vi "Actor Core.vi"(8 "error in":errorcluster, 11 "Create Test Node View in":refnum<class "Edit Test Node View.lvclass">) -> (0 "error out":errorcluster, 3 "Actor out":refnum<class "Actor.lvclass">)   [LabVIEW 2013, in "Edit Test Node View.lvlib" / "Edit Test Node View.lvclass"]
doc: "(<B>Filename</B>: Actor Framework.lvlib:Actor.lvclass:Actor Core.vi)\n\nReceives messages to the actor, reacts to them, and initiates any error handling that may shut the actor down.\n\nDescendant classes may override this VI to append parallel tasks for the actor to complete while it handles messages. Overrides use the Call Parent Method node."
uses:
  Edit Test Node View.lvclass
  <vilib>/ActorFramework/Actor/Actor.lvclass
  Resources/UI Controls/Textbox.ctl
  <vilib>/ActorFramework/Actor/Actor.lvclass/Actor.ctl
  <vilib>/ActorFrameworkMVC/View Actor/View Actor.lvclass
  <vilib>/ActorFramework/Message Enqueuer/Message Enqueuer.lvclass/Message Enqueuer.ctl
  Edit Test Node View.lvclass/Edit Test Node View.ctl
  Models/Edit Test Node Model Messages/Set Item Configurations Msg/Set Item Configurations Msg.lvclass/Set Item Configurations Msg.ctl
  <vilib>/Utility/miscctls.llb/LVPositionTypeDef.ctl
  <vilib>/ActorFrameworkMVC/UI Controller Messages/Move Subpanel Msg/Move Subpanel Msg.lvclass/Move Subpanel Msg.ctl
  <vilib>/ActorFrameworkMVC/UI Controller Messages/Insert Subpanel Msg/Insert Subpanel Msg.lvclass/Insert Subpanel Msg.ctl
  <vilib>/ActorFramework/Message Enqueuer/Init from Existing Queue.vi
  <vilib>/ActorFramework/Message Enqueuer/Enqueue.vi
  <vilib>/ActorFramework/Message Priority Queue/Priority Enqueue.vi
  <vilib>/ActorFramework/Message Enqueuer/Message Enqueuer.lvclass
  Models/Edit Test Node Model Messages/Set Item Configurations Msg/Set Item Configurations Msg.lvclass
  Models/Edit Test Node Model Messages/Load Test Node Msg/Load Test Node Msg.lvclass
  Models/Edit Test Node Model Messages/Save Test Node Msg/Save Test Node Msg.lvclass
  <vilib>/ActorFrameworkMVC/UI Controller Messages/Move Subpanel Msg/Move Subpanel Msg.lvclass
  <vilib>/ActorFrameworkMVC/UI Controller Messages/Insert Subpanel Msg/Insert Subpanel Msg.lvclass
  Models/Test Node Model Messages/Preview Test Node Msg/Preview Test Node Msg.lvclass
  Models/Test Node Model Messages/Update Tiles Info Msg/Update Tiles Info Msg.lvclass
  Models/Test Node Model Messages/Update Previous Button Visibility Msg/Update Previous Button Visibility Msg.lvclass
  Models/Test Node Model Messages/Update Next Button Visibility Msg/Update Next Button Visibility Msg.lvclass
  Common/File IO/File IO.lvlib
  <vilib>/ActorFrameworkMVC/View Actor Messages/Get Model Enqueuer Msg/Get Model Enqueuer Msg.lvclass
  <vilib>/ActorFrameworkMVC/UI Controller Messages/Get Model Actor Enqueuer Msg/Get Model Actor Enqueuer Msg.lvclass
panel:
  in  "Cancel":bool
  in  "Save":bool
  out "Tab Control":enum32{"Basic Info"}(tab)
  in  "Node Description":string caption="测试节点描述："
  in  "Node Name":string caption="测试节点名称："
  in  "Node Abbreviation":string caption="测试节点英文简写："
  in  "Node Type":u16(ring) caption="测试节点类型：" items=["模拟电压", "模拟电流", "数字", "RS232", "RS485"]
  in  "Node MAC":T1 caption="测试节点MAC"
  # "编辑测试节点"
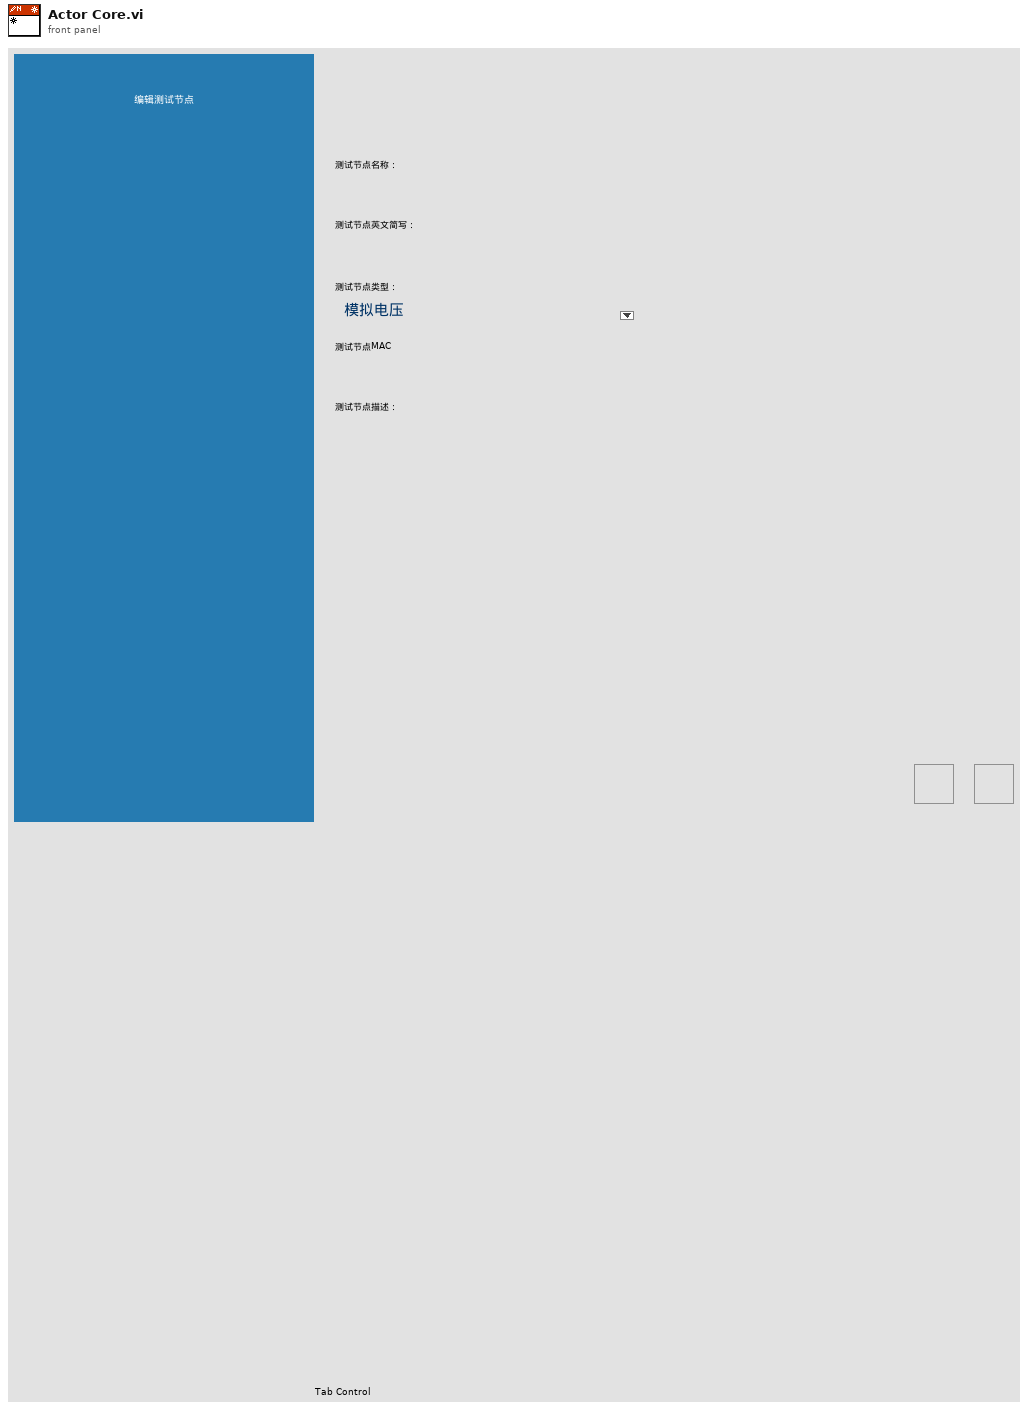
[diagram p1: front panel]
types:
  T1 = typedef "Textbox.ctl" = string
  T2 = typedef "Edit Test Node View.lvlib/Edit Test Node View.lvclass/Events.ctl" = cluster{"Reinitialize All":refnum<user-event>}
  T3 = typedef "LVPositionTypeDef.ctl" = cluster{"Left":i32, "Top":i32}
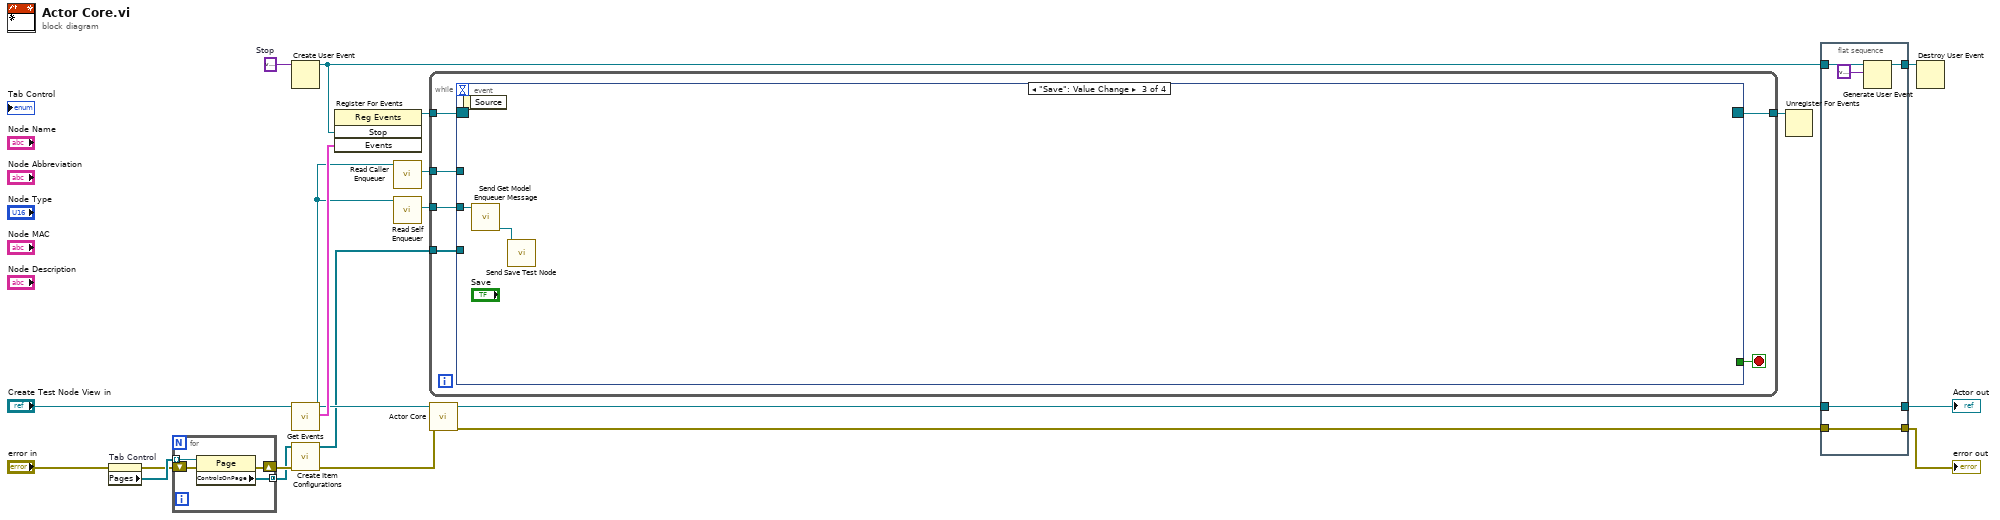
[diagram p0: block diagram]
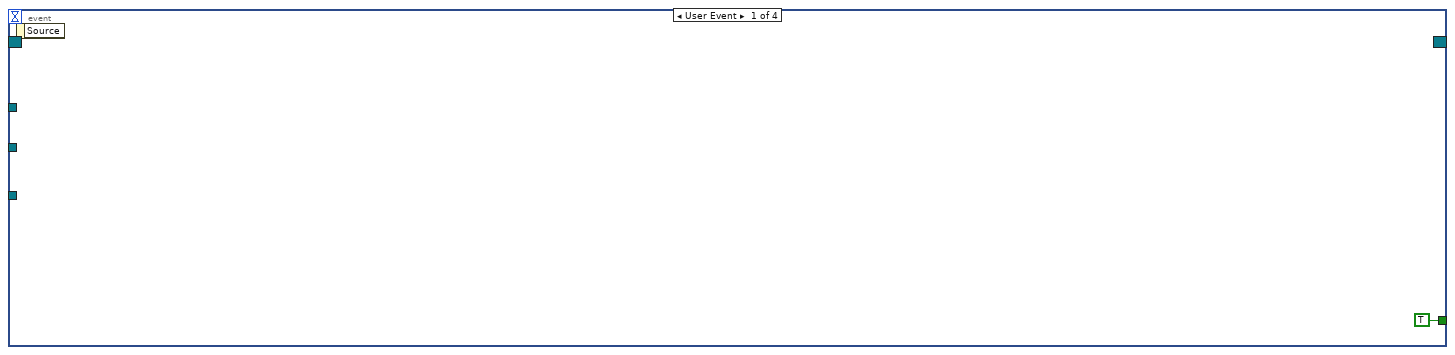
[diagram p2: hidden frame]
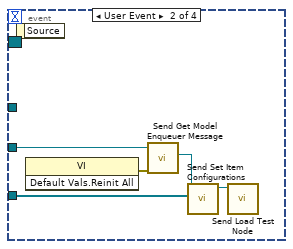
[diagram p3: hidden frame]
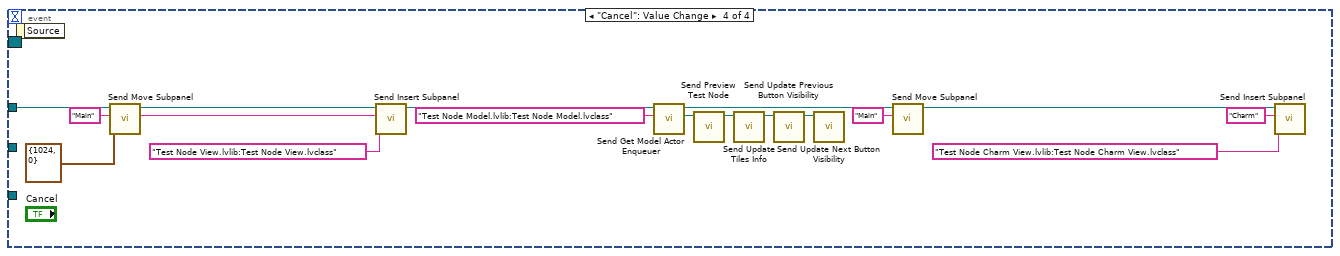
[diagram p4: hidden frame]
diagram:
  w21 = variant  # Stop
  n1 = property on="Tab Control" class="TabCtl (strict)"(error in="error in") -> (error out=w10:errorcluster, "Pages"=w11:refnum<vi>[])  [unwired: 1 in, 1 out]
  n2 = for {
    tunnel: w11 -> [w25] mode=indexing
    tunnel: [w24] -> w8 mode=concatenating
    shift-right: [w22] -> w9
    shift-left: w10 -> [w23]
    n3 = property class="Page"(reference=w25, error in=w23) -> (error out=w22:errorcluster, "ControlsOnPage"=w24:refnum<vi>[])  [unwired: 1 out]
  }
  n4 = Create User Event(user event datatype=w21) -> (user event=w14:refnum<user-event>)  [unwired: 1 in, 1 out]
  n5 = call "Get Events.vi"("Create Test Node View in"="Create Test Node View in") -> ("Events"=w13:T2, "Create Test Node View out"=w4:refnum<class "Edit Test Node View.lvclass">)  [unwired: 9 in]
  n6 = call "Create Item Configurations.vi"("error in (no error)"=w9, "Controls References"=w8) -> ("error out"=w3:errorcluster, "Item Configurations"=w1:refnum<class "Item Configuration.lvclass">[])  [unwired: 8 in]
  n7 = register-events(w14, w13) -> (reference out=w15:refnum<event-registration>)  [unwired: 2 in, 1 out]
  n8 = call <vilib>:"Read Caller Enqueuer.vi"("Actor"=w4) -> ("Caller Enqueuer"=w6:refnum<class "Message Enqueuer.lvclass">)  [unwired: 10 in]
  n9 = call <vilib>:"Read Self Enqueuer.vi"("Actor"=w4) -> ("Self Enqueuer"=w5:refnum<class "Message Enqueuer.lvclass">)  [unwired: 10 in]
  n10 = while {
    tunnel: [w31] -> w12
    tunnel: w15 -> [w29]
    tunnel: w6 -> [w28]
    tunnel: w5 -> [w27]
    tunnel: w1 -> [w26]
    stop <- w30 stop-if-true
    n11 = event shown="[2] \"Save\": Value Change" {
      selector: w29 -> [_ _ _ _]
      dyn-events: [_ _ _ _] -> w31
      timeout: _ -> [_ _ _ _]
      tunnel: [TRUE _ _ _] -> w30
      tunnel: w28 -> [_ _ _ w41]
      tunnel: w27 -> [_ w34 w38 _]
      tunnel: w26 -> [_ w33 _ _]
      event User Event {
        n12 = event-data() -> ()  [unwired: 1 in, 1 out]
      }
      event User Event {
        n13 = event-data() -> ()  [unwired: 1 in, 1 out]
        n14 = invoke class="VI" method="Default Vals.Reinit All"() -> (error out=w37:errorcluster)  [unwired: 3 in, 2 out]
        n15 = call <vilib>:"Send Get Model Enqueuer Message.vi"("error in (no error)"=w37, "Message Enqueuer in"=w34) -> ("Reply"=w36:refnum<class "Message Enqueuer.lvclass">)  [unwired: 6 in, 3 out]
        n16 = call "Send Set Item Configurations.vi"("Item Configurations"=w33, "Message Enqueuer"=w36) -> ("Message Enqueuer out"=w35:refnum<class "Message Enqueuer.lvclass">)  [unwired: 8 in, 1 out]
        n17 = call "Send Load Test Node.vi"("Message Enqueuer"=w35) -> ()  [unwired: 9 in, 2 out]
      }
      event "Save": Value Change {
        n18 = event-data() -> ()  [unwired: 1 in, 1 out]
        n19 = call <vilib>:"Send Get Model Enqueuer Message.vi"("Message Enqueuer in"=w38) -> ("Reply"=w39:refnum<class "Message Enqueuer.lvclass">)  [unwired: 7 in, 3 out]
        n20 = call "Send Save Test Node.vi"("Message Enqueuer"=w39) -> ()  [unwired: 9 in, 2 out]
      }
      event "Cancel": Value Change {
        w52 = "Main" ("Subpanel Name")
        n21 = event-data() -> ()  [unwired: 1 in, 1 out]
        n22 = call <vilib>:"Send Move Subpanel.vi"("Position (0,0)"=T3 {"Left"=1024, "Top"=0}, "Subpanel Name"=w52, "Message Enqueuer"=w41) -> ("Message Enqueuer out"=w55:refnum<class "Message Enqueuer.lvclass">)  [unwired: 7 in, 1 out]
        n23 = call <vilib>:"Send Insert Subpanel.vi"("View Name"="Test Node View.lvlib:Test Node View.lvclass" ("Subpanel Name"), "Subpanel Name"=w52, "Message Enqueuer"=w55) -> ("Message Enqueuer out"=w50:refnum<class "Message Enqueuer.lvclass">)  [unwired: 7 in, 1 out]
        n24 = call <vilib>:"Send Get Model Actor Enqueuer.vi"("Model Name"="Test Node Model.lvlib:Test Node Model.lvclass", "Message Enqueuer in"=w50) -> ("Reply"=w40:refnum<class "Message Enqueuer.lvclass">, "Message Enqueuer out"=w49:refnum<class "Message Enqueuer.lvclass">)  [unwired: 6 in, 2 out]
        n25 = call "Send Preview Test Node.vi"("Message Enqueuer"=w40) -> ("Message Enqueuer out"=w47:refnum<class "Message Enqueuer.lvclass">)  [unwired: 9 in, 1 out]
        n26 = call "Send Update Tiles Info.vi"("Message Enqueuer"=w47) -> ("Message Enqueuer out"=w46:refnum<class "Message Enqueuer.lvclass">)  [unwired: 9 in, 1 out]
        n27 = call "Send Update Previous Button Visibility.vi"("Message Enqueuer"=w46) -> ("Message Enqueuer out"=w45:refnum<class "Message Enqueuer.lvclass">)  [unwired: 9 in, 1 out]
        n28 = call "Send Update Next Button Visibility.vi"("Message Enqueuer"=w45) -> ()  [unwired: 9 in, 2 out]
        n29 = call <vilib>:"Send Move Subpanel.vi"("Subpanel Name"="Main", "Message Enqueuer"=w49) -> ("Message Enqueuer out"=w44:refnum<class "Message Enqueuer.lvclass">)  [unwired: 8 in, 1 out]
        n30 = call <vilib>:"Send Insert Subpanel.vi"("View Name"="Test Node Charm View.lvlib:Test Node Charm View.lvclass", "Subpanel Name"="Charm", "Message Enqueuer"=w44) -> ()  [unwired: 7 in, 2 out]
      }
    }
  }
  n31 = call-parent "Actor Core.vi"("error in"=w3, "View Actor in"=w4) -> ("error out"=w18:errorcluster, "Actor out"=w19:refnum<class "Actor.lvclass">)  [unwired: 8 in]
  n32 = Unregister For Events(event registration refnum=w12) -> ()  [unwired: 1 in, 1 out]
  n33 = flat-sequence "Generate a stop event when the actor core stopped." {
    tunnel: w14 -> [w60]
    tunnel: [w58] -> w20
    tunnel: w19 -> [w57]
    tunnel: w18 -> [w56]
    tunnel: [w57] -> w17
    tunnel: [w56] -> w16
    frame #0 {
      n34 = Generate User Event(user event=w60, event data cluster=variant ("event data")) -> (user event out=w58:refnum<user-event>)  [unwired: 2 in, 1 out]
    }
  }
  n35 = Destroy User Event(user event=w20) -> ()  [unwired: 1 in, 1 out]
  "error out" <- w16
  "Actor out" <- w17
